vi "Cleanup.vi"(8 "error in (no error)":errorcluster, 11 "Request in":refnum<class "Request.lvclass">) -> (0 "error out":errorcluster)   [LabVIEW 2020, in "HTTP Utils.lvlib" / "Request.lvclass"]
doc: "Cleans up any resources allocated for the request such as file uploads. To ensure future compatibilty always call this VI when finishing a request to prevent issues as functionality is added in the future.\n\nThis does not cleanup / close the underlying connection. The connection will remain in a valid state (assuming the connection wasn't previously closed) for reuse with features such as Connection: keep-alive"
uses:
  Request.lvclass
  Request.lvclass/Request.ctl
  FormField/FormField.lvclass
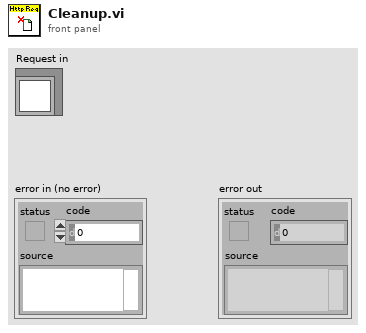
[diagram p1: front panel]
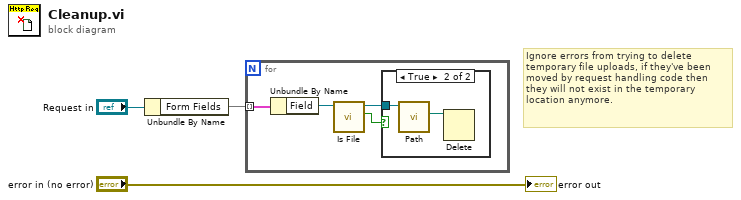
[diagram p0: block diagram]
diagram:
  # "Ignore errors from trying to delete temporary file uploads, if they've been moved by request handling code then they will not exist in the temporary location anymore."
  n1 = Unbundle By Name("Request in") -> ("Form Fields"=w1:map{string, refnum<class "FormField.lvclass">})
  n2 = for {
    tunnel: w1 -> [w7] mode=indexing
    n3 = Unbundle By Name(w7) -> ("Field"=w6:refnum<class "FormField.lvclass">)
    n4 = call "Is File.vi"("FormField in"=w6) -> ("Is File?"=w4:bool, "FormField out"=w5:refnum<class "FormField.lvclass">)  [unwired: 8 in, 1 out]
    n5 = case shown="True" w4 {
      tunnel: w5 -> [_ w9]
      frame False {
      }
      frame True {
        n6 = call "Path.vi"("FormField in"=w9) -> ("Path"=w8:path)  [unwired: 8 in, 2 out]
        n7 = Delete(path (use dialog)=w8) -> ()  [unwired: 4 in, 3 out]
      }
    }
  }
  "error out" <- "error in (no error)"
